vi "Post-BuildCreateFileVersionTxt.vi"(5 "Files Generated by Build":path[](array[path]), 6 "Top Level/Always Included VIs":path[](array[path]), 7 "Destination Path":path, 8 "error in (no error)":errorcluster, 9 "Target Name":string, 10 "Build Specification Name":string, 11 "Project Path":path) -> (0 "error out":errorcluster)   [LabVIEW 2011, in "Medimatic.lvlib"]
uses:
  Medimatic.lvlib
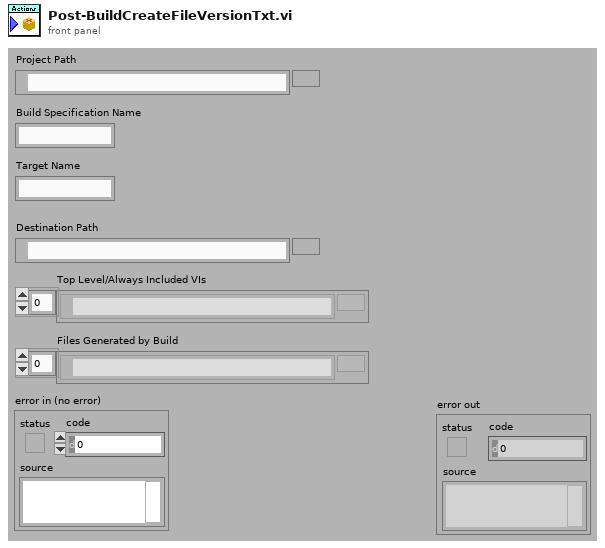
[diagram p1: front panel]
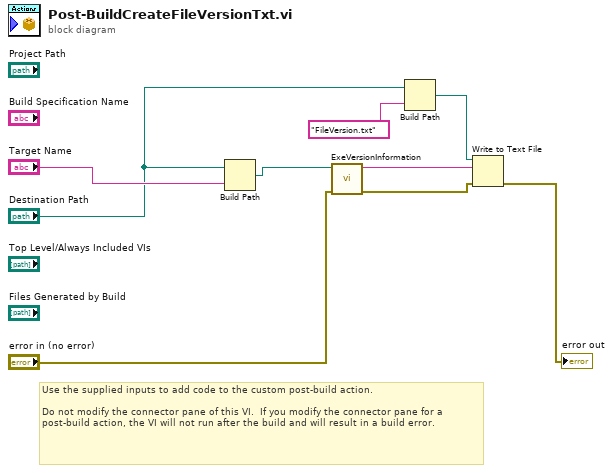
[diagram p0: block diagram]
diagram:
  # "Use the supplied inputs to add code to the custom post-build action.\n\nDo not modify the connector pane of this VI.  If you modify the connector pane for a post-build action, the VI will not run after the build and will result in a build error."
  n1 = Build Path(base path="Destination Path", name or relative path="Target Name") -> (appended path=w5:path)
  n2 = call "ExeVersionInformation.vi"("error in (no error)"="error in (no error)", "path"=w5) -> ("error out"=w9:errorcluster, "FileVersion"=w6:string)  [unwired: 8 in]
  n3 = Build Path(base path="Destination Path", name or relative path="FileVersion.txt") -> (appended path=w8:path)
  n4 = Write to Text File(file (use dialog)=w8, text=w6, error in=w9) -> (error out=→"error out":errorcluster)  [unwired: 1 in, 2 out]
